vi "get Requested Resources property.vi"(8 "error in (no error)":errorcluster, 11 "Item Ref in":T1 format="%.0x") -> (0 "error out":errorcluster, 2 "Requested Resources":T2, 3 "Item Ref out":T1 format="%.0x")   [LabVIEW 2016, in "FPGA RM System Definition API.lvlib"]
uses:
  FPGA RM System Definition API.lvlib
  <vilib>/NI Veristand/Custom Device API/Custom Device Item Ref.ctl
  Shared/FPGA Configuration Classes/Datatype Group/Requested Resources.ctl
  Shared/Types/Requested Resource.ctl
  Shared/Types/Channel Type.ctl
  <vilib>/NI Veristand/Custom Device API/Get Item Property (Variant).vi
  <vilib>/NI VeriStand/Custom Device API/Custom Device API.lvlib
  Shared/FPGA RM Shared API.lvlib
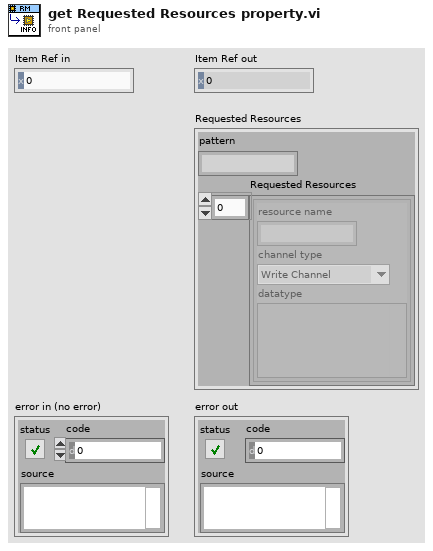
[diagram p1: front panel]
types:
  T1 = typedef "Custom Device API.lvlib/Custom Device Item Ref.ctl" = u64
  T2 = typedef "FPGA RM Shared API.lvlib/Requested Resources.ctl" = cluster{"pattern":string, "Requested Resources":T3[]}
  T3 = typedef "FPGA RM Shared API.lvlib/Requested Resource.ctl" = cluster{"resource name":string, "channel type":T4, "datatype":variant}
  T4 = typedef "FPGA RM Shared API.lvlib/Channel Type.ctl" = enum16{"Write Channel", "Read Channel", "Write Waveform", "Read Waveform"}
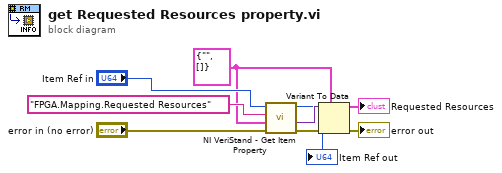
[diagram p0: block diagram]
diagram:
  w6 = T2 {"pattern"="", "Requested Resources"=[]} ("Requested Resources")
  n1 = call-poly <vilib>:"NI VeriStand - Get Item Property.vi"("error in (no error)"="error in (no error)", "Default Value"=w6, "Property Name"="FPGA.Mapping.Requested Resources", "Item Ref in"="Item Ref in") -> ("error out"=w5:errorcluster, "Value"=w7:variant, "Item Ref out"=→"Item Ref out":T1)  [unwired: 4 in, 1 out]
  n2 = Variant To Data(error in=w5, type=w6, Variant=w7) -> (data=→"Requested Resources":T2, error out=→"error out":errorcluster)
